vi "getEncoderPosition.vi"(8 "error in (no error)":errorcluster, 11 "AdaFruit-Seesaw in":refnum<class "AdaFruit-Seesaw.lvclass">) -> (0 "error out":errorcluster, 2 "Position":i32, 3 "AdaFruit-Seesaw out":refnum<class "AdaFruit-Seesaw.lvclass">)   [LabVIEW 2020, in "CTI-Peripheral.lvlib" / "AdaFruit-Seesaw.lvclass"]
uses:
  AdaFruit-Seesaw.lvclass
  Private/SeeSawENCODERFunctions.ctl
  Private/SeeSawBaseAddresses.ctl
  AdaFruit-Seesaw.lvclass/AdaFruit-Seesaw.ctl
  CTI/I2C Connection/I2C Connection.lvclass/I2C Connection.ctl
  CTI/Session/I2C Write Data.vi
  CTI/Session/I2C Read Data.vi
  CTI/I2C Connection/I2C Connection.lvclass
panel:
  out "Data":string
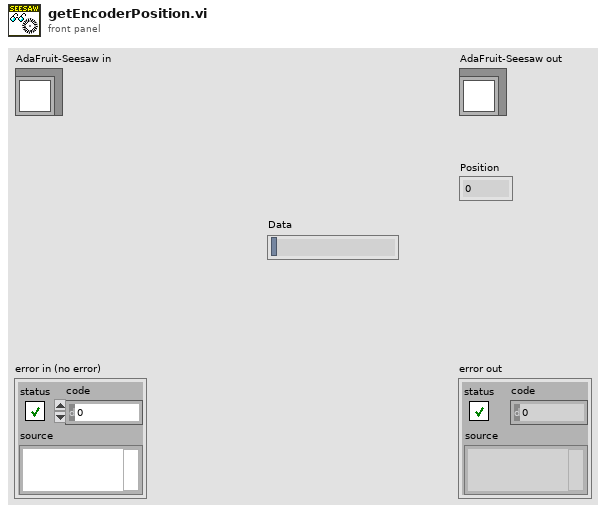
[diagram p1: front panel]
types:
  T1 = typedef "CTI-Peripheral.lvlib/AdaFruit-Seesaw.lvclass/SeeSawBaseAddresses.ctl" = u8
  T2 = typedef "CTI-Peripheral.lvlib/AdaFruit-Seesaw.lvclass/SeeSawENCODERFunctions.ctl" = u8
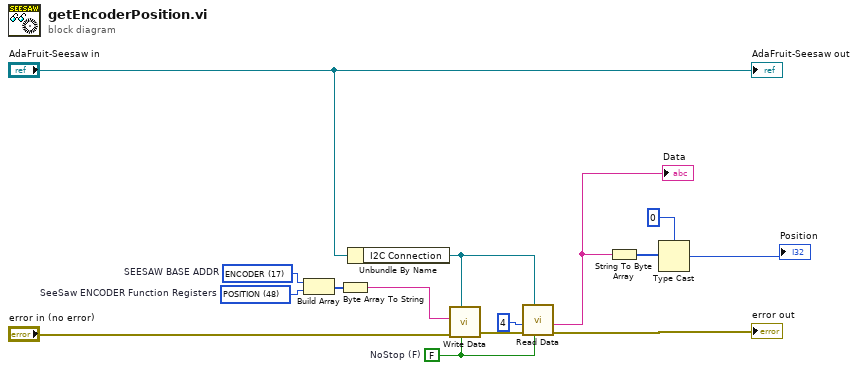
[diagram p0: block diagram]
diagram:
  w8 = FALSE  # NoStop (F)
  w15 = T1 17 items=["STATUS"=0, "GPIO"=1, "SERCOM0"=2, "TIMER"=8, "ADC"=9, "DAC"=10, "INTERUPT"=11, "DAP"=12, "EEPROM"=13, "NEOPIXEL"=14, "TOUCH"=15, "KEYPAD"=16, "ENCODER"=17, "SPECTRUM"=18]  # SEESAW BASE ADDR
  w14 = T2 48 items=["STATUS"=0, "INTENSET"=16, "INTENCLR"=32, "POSITION"=48, "DELTA"=64]  # SeeSaw ENCODER Function Registers
  n1 = Build Array(w15, w14) -> (w13:T2[])
  n2 = Byte Array To String(unsigned byte array=w13) -> (string=w7:string)
  n3 = Unbundle By Name("AdaFruit-Seesaw in") -> ("I2C Connection"=w9:refnum<class "I2C Connection.lvclass">)
  n4 = call "Write Data.vi"("NoStop (F)"=w8, "I2C Connection"=w9, "error in (no error)"="error in (no error)", "Data"=w7) -> ("error out"=w12:errorcluster)  [unwired: 7 in]
  n5 = call "Read Data.vi"("NoStop (F)"=w8, "I2C Connection"=w9, "error in (no error)"=w12, "Len"=u8 4 ("Read Len")) -> ("error out"=→"error out":errorcluster, "Data"=w4:string)  [unwired: 6 in]
  "Data" <- w4
  n6 = String To Byte Array(string=w4) -> (unsigned byte array=w2:u8[])
  n7 = Type Cast(type=0 ("Position"), x=w2) -> (*(type *) &x=→"Position":i32)
  "AdaFruit-Seesaw out" <- "AdaFruit-Seesaw in"
